vi "TCL Baseline Lookup.vi"(2 "Fragments Desired":string[](array[string]), 3 "Events Requested":i32[](array[numeric])) -> (0 "Data":string[][](array[string]), 1 "Fragments Returned":string[](array[string]))   [LabVIEW 2009]
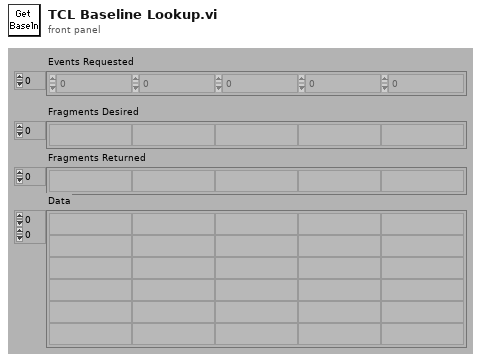
[diagram p1: front panel]
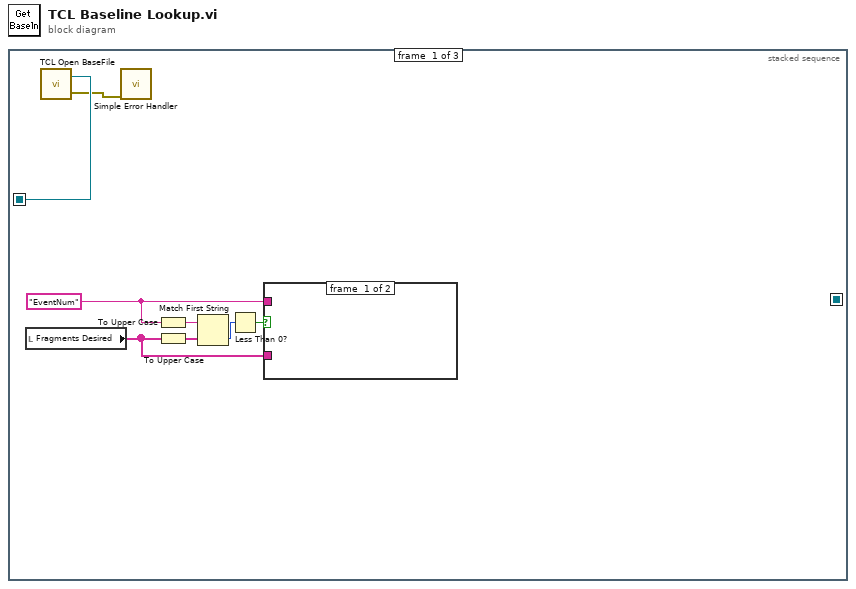
[diagram p0: block diagram]
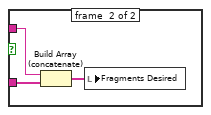
[diagram p2: hidden frame]
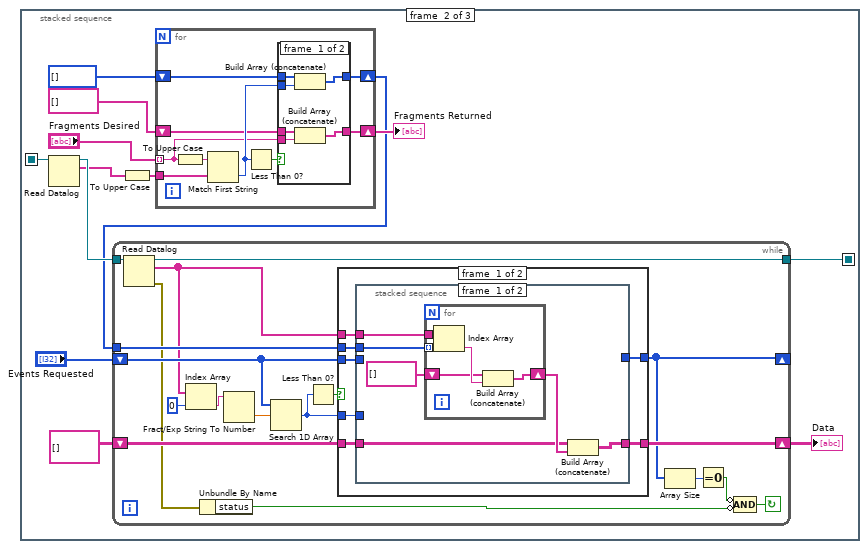
[diagram p3: hidden frame]
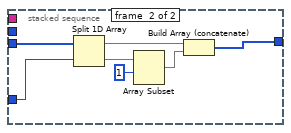
[diagram p4: hidden frame]
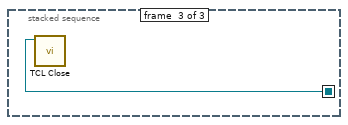
[diagram p7: hidden frame]
diagram:
  n1 = stacked-sequence {
    seq-local: [w2 _ _] -> [_ w18 _]
    seq-local: [_ w15 _] -> [_ _ w87]
    frame #0 {
      w4 = "EventNum"
      n2 = local read "Fragments Desired"() -> (w3:string[])
      n3 = call "TCL Open BaseFile.vi"() -> ("error out"=w1:errorcluster, "Event File Refnum"=w2:refnum<k1>)
      n4 = call <vilib>:"Simple Error Handler.vi"("error in (no error)"=w1) -> ()  [unwired: 4 in, 5 out]
      n5 = To Upper Case(1:w4) -> (0:w8:string)
      n6 = To Upper Case(1:w3) -> (0:w7:string[])
      n7 = Match First String(2:w7, 3:w8) -> (0:w6:i32)  [unwired: 1 out]
      n8 = Less Than 0?(x=w6) -> (x < 0?=w5:bool)
      n9 = case shown="True" w5 {
        tunnel: w4 -> [_ w11]
        tunnel: w3 -> [_ w10]
        frame #0 {
        }
        frame #1 {
          n10 = Build Array (concatenate)(w11, w10) -> (w9:string[])
          n11 = local write "Fragments Desired"(w9) -> ()
        }
      }
    }
    frame #1 {
      n12 = Read Datalog(7:w18) -> (2:w12:string[], 3:w17:refnum<k1>)  [unwired: 2 in, 1 out]
      n13 = To Upper Case(1:w12) -> (0:w23:string[])
      n14 = for {
        tunnel: w23 -> [w78]
        tunnel: "Fragments Desired" -> [w71] mode=indexing
        shift-right: [w74] -> w13
        shift-left: i32[] [] -> [w75]
        shift-right: [w72] -> w22
        shift-left: string[] [] -> [w73]
        n15 = To Upper Case(1:w71) -> (0:w70:string)
        n16 = Match First String(2:w78, 3:w70) -> (0:w77:i32)  [unwired: 1 out]
        n17 = Less Than 0?(x=w77) -> (x < 0?=w76:bool)
        n18 = case shown="False" w76 {
          tunnel: w77 -> [w83 _]
          tunnel: w75 -> [w84 w86]
          tunnel: [w82 w86] -> w74
          tunnel: w73 -> [w81 w85]
          tunnel: [w80 w85] -> w72
          tunnel: w71 -> [w79 _]
          frame #0 {
            n19 = Build Array (concatenate)(w84, w83) -> (w82:i32[])
            n20 = Build Array (concatenate)(w81, w79) -> (w80:string[])
          }
          frame #1 {
          }
        }
      }
      "Fragments Returned" <- w22
      n21 = while {
        tunnel: w13 -> [w35]
        shift-left: string[][] [] ("Data") -> [w33]
        shift-right: [w32] -> w14
        tunnel: [w41] -> w15
        tunnel: w17 -> [w42]
        shift-left: "Events Requested" -> [w34]
        shift-right: [w31] -> _
        stop <- w30 continue-if-true
        n22 = Read Datalog(7:w42) -> (0:w26:errorcluster, 2:w27:string[], 3:w41:refnum<k1>)  [unwired: 2 in]
        n23 = Index Array(array=w27, index=0) -> (element=w39:string)
        n24 = Unbundle By Name(w26) -> ("status"=w25:bool)
        n25 = Fract/Exp String To Number(string=w39) -> (number=w38:dbl)  [unwired: 3 in, 1 out]
        n26 = Search 1D Array(1D array=w34, element=w38) -> (index of element=w37:i32)  [unwired: 1 in]
        n27 = Less Than 0?(x=w37) -> (x < 0?=w36:bool)
        n28 = case shown="False" w36 {
          tunnel: w37 -> [w47 _]
          tunnel: w27 -> [w48 _]
          tunnel: w35 -> [w49 _]
          tunnel: w34 -> [w44 w68]
          tunnel: w33 -> [w46 w69]
          tunnel: [w45 w69] -> w32
          tunnel: [w43 w68] -> w31
          frame #0 {
            n29 = stacked-sequence {
              tunnel: w49 -> [w55 _]
              tunnel: w48 -> [w54 _]
              tunnel: w47 -> [_ w66]
              tunnel: w46 -> [w51 _]
              tunnel: [w50 _] -> w45
              tunnel: w44 -> [_ w67]
              tunnel: [_ w61] -> w43
              frame #0 {
                n30 = for {
                  tunnel: w55 -> [w59] mode=indexing
                  tunnel: w54 -> [w60]
                  shift-right: [w56] -> w52
                  shift-left: string[] [] -> [w57]
                  n31 = Index Array(array=w60, index=w59) -> (element=w58:string)
                  n32 = Build Array (concatenate)(w57, w58) -> (w56:string[])
                }
                n33 = Build Array (concatenate)(w51, w52) -> (w50:string[][])
              }
              frame #1 {
                n34 = Split 1D Array(array=w67, index=w66) -> (first subarray=w65:i32[], second subarray=w63:i32[])
                n35 = Array Subset(array=w63, index=1) -> (w64:i32[])  [unwired: 1 in]
                n36 = Build Array (concatenate)(w65, w64) -> (w61:i32[])
              }
            }
          }
          frame #1 {
          }
        }
        n37 = Array Size(array=w31) -> (size(s)=w29:i32)
        n38 = Equal To 0?(x=w29) -> (x = 0?=w28:bool)
        n39 = Compound Arithmetic op=AND(invert w28, invert w25) -> (w30:bool)
      }
      "Data" <- w14
    }
    frame #2 {
      n40 = call "TCL Close.vi"("Event File Refnum"=w87) -> ()  [unwired: 3 in]
    }
  }
